vi "Initialize.vi"(8 "error in (no error)":errorcluster, 11 "direct handler in":refnum<class "Direct Handler.lvclass">) -> (0 "error out":errorcluster, 3 "direct handler out":refnum<class "Direct Handler.lvclass">)   [LabVIEW 2018, in "GLog.lvlib" / "Direct Handler.lvclass"]
uses:
  Direct Handler.lvclass
  formatting_handler_interface/Formatting Handler.lvclass
panel:
  # "Connector Pane"
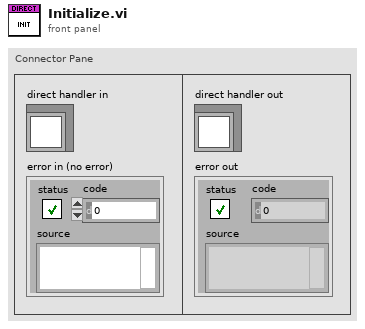
[diagram p1: front panel]
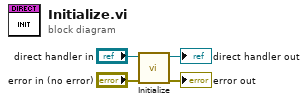
[diagram p0: block diagram]
diagram:
  n1 = call-parent "Initialize.vi"("error in (no error)"="error in (no error)", "handler in"="direct handler in") -> ("error out"=→"error out":errorcluster, "handler out"=→"direct handler out":refnum<class "Direct Handler.lvclass">)  [unwired: 8 in]
